vi "State Open Libraries.vi"(8 "error in (no error)":errorcluster, 11 "Lua in":refnum<class "Lua.lvclass">) -> (0 "error out":errorcluster, 3 "Lua out":refnum<class "Lua.lvclass">)   [LabVIEW 2020, in "Lua for LabVIEW.lvlib" / "Lua.lvclass"]
doc: "Opens all standard Lua libraries into the given state."
uses:
  Lua.lvclass
  Lua.lvclass/Lua.ctl
  lib/lua.dll/lua.dll.lvlib
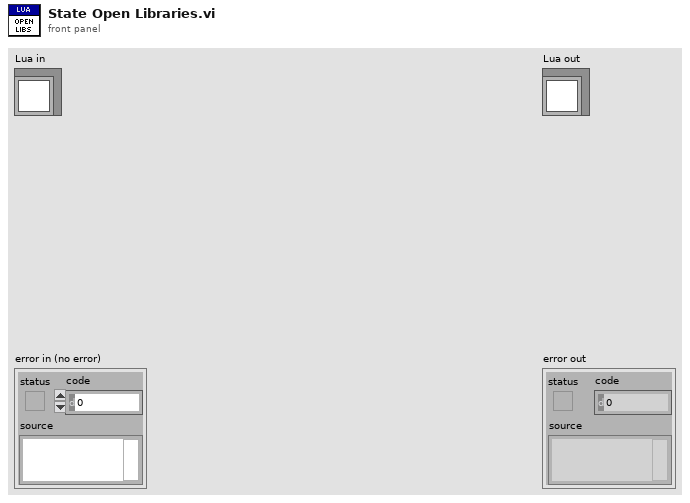
[diagram p1: front panel]
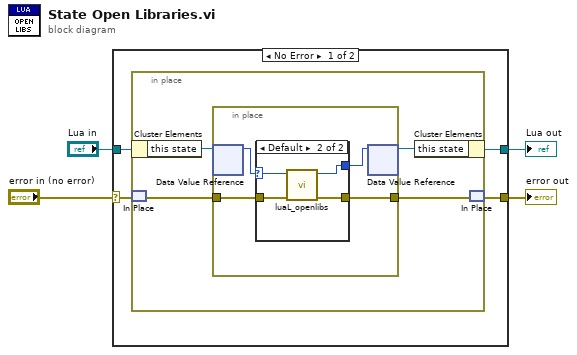
[diagram p0: block diagram]
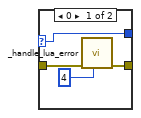
[diagram p2: hidden frame]
diagram:
  n1 = case shown="No Error" "error in (no error)" {
    selector: "error in (no error)" -> [w5 w26]
    tunnel: [w6 w26] -> w1
    tunnel: [w7 w25] -> w4
    tunnel: "Lua in" -> [w8 w25]
    frame No Error {
      n2 = in-place {
        n3 = in-place-cluster #1(w8) -> ("this state"=w10:refnum<data-value>)
        n4 = in-place-match #2(w5) -> (w12:errorcluster)
        n5 = in-place {
          in-place-border: w12 -> [w16]
          in-place-border: [w15] -> w11
          n6 = in-place-dvr #3(w10) -> (w14:u64)  [unwired: 1 out]
          n7 = case shown="Default" w14 {
            selector: w14 -> [w20 w24]
            tunnel: [w20 w23] -> w13
            tunnel: w16 -> [w17 w21]
            tunnel: [w18 w22] -> w15
            frame 0 {
              n8 = call "_handle_lua_error.vi"("lua status"=4 ("lua_load errcode"), "error in (no error)"=w17) -> ("error out"=w18:errorcluster)  [unwired: 9 in]
            }
            frame Default {
              n9 = call "luaL_openlibs.vi"("error in (no error)"=w21, "lua_state_p"=w24) -> ("error out"=w22:errorcluster, "lua_state_p out"=w23:u64)  [unwired: 8 in]
            }
          }
          n10 = in-place-dvr #3(w13) -> (w9:refnum<data-value>)  [unwired: 1 out]
        }
        n11 = in-place-cluster #1("this state"=w9) -> (w7:refnum<class "Lua.lvclass">)
        n12 = in-place-match #2(w11) -> (w6:errorcluster)
      }
    }
    frame Error {
    }
  }
  "error out" <- w1
  "Lua out" <- w4
